vi "Check Expiration.vi"(0 "Vector Charact Result Accessor in":refnum<class "Vector Charact Result Accessor.lvclass">, 11 "error in":errorcluster) -> (4 "Vector Charact Result Accessor out":refnum<class "Vector Charact Result Accessor.lvclass">, 6 "Expired?":bool, 15 "error out":errorcluster)   [LabVIEW 2023, in "RFFixtureCharact.Public.lvlib" / "Vector Charact Result Accessor.lvclass"]
uses:
  Vector Charact Result Accessor.lvclass
  C:/rfcal/AuxTools/STSRFFixtureCharactUtility/Source/Code Modules/Fixture/RMM/Charact Result Accessor/Base/Charact Result Accessor.lvclass
  <vilib>/addons/_RFCalAndCharactDatabase/NI_RFCalAndCharact_Database_API.lvlibp/Characterization/Controls/Type.ctl
  Vector Charact Result Accessor.lvclass/Vector Charact Result Accessor.ctl
  <vilib>/addons/_RFCalAndCharactDatabase/NI_RFCalAndCharact_Database_API.lvlibp/Characterization/Characterization.lvlib
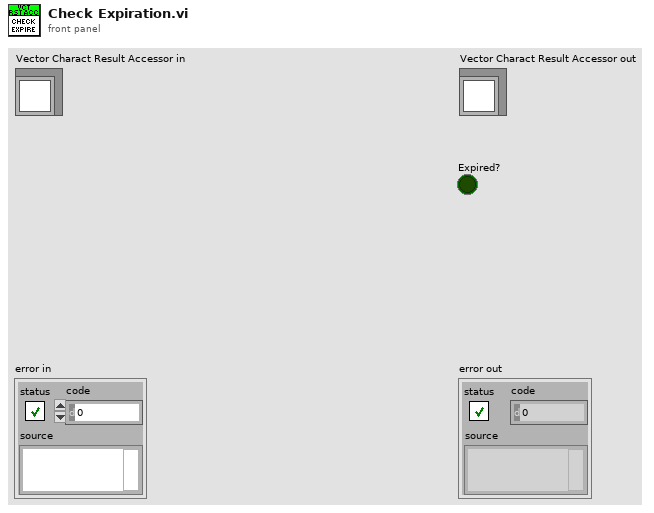
[diagram p1: front panel]
types:
  T1 = typedef "NI_RFCalAndCharact_Database_API.lvlibp/Characterization.lvlib/Type.ctl" = u16
  T2 = typedef "NI_RFCalAndCharact_Database_API.lvlibp/Characterization.lvlib/Path Handle.ctl" = refnum<k24>
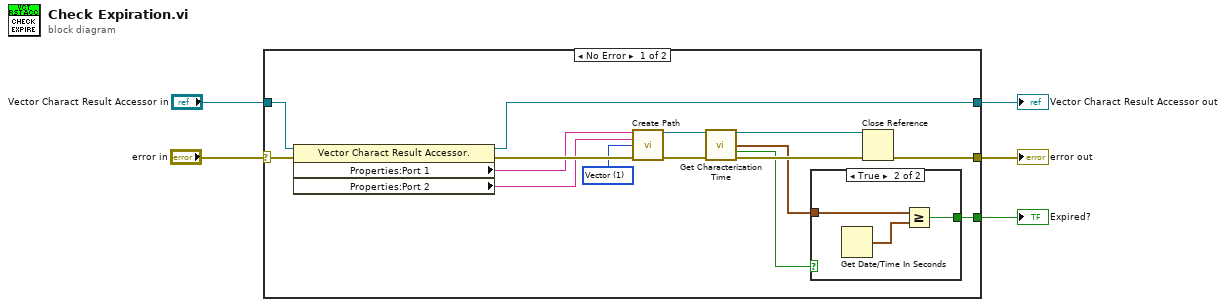
[diagram p0: block diagram]
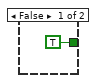
[diagram p2: hidden frame]
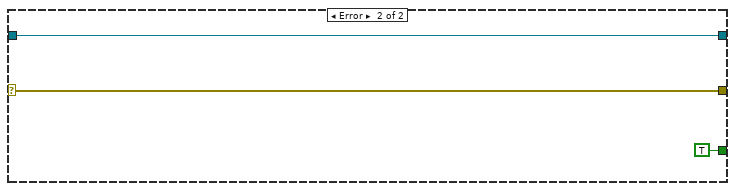
[diagram p3: hidden frame]
diagram:
  n1 = case shown="No Error" "error in" {
    selector: "error in" -> [w15 w26]
    tunnel: "Vector Charact Result Accessor in" -> [w16 w27]
    tunnel: [w10 w27] -> w2
    tunnel: [w9 w26] -> w4
    tunnel: [w6 TRUE] -> w3
    frame No Error {
      w17 = T1 1 items=["Scalar", "Vector"] ("Type")
      n2 = property class="Vector Charact Result Accessor."(reference=w16, error in=w15) -> (reference out=w10:refnum<class "Vector Charact Result Accessor.lvclass">, error out=w20:errorcluster, "Properties:Port 1"=w18:string, "Properties:Port 2"=w19:string)
      n3 = call <vilib>:"Create Path.vi"("Port 1"=w18, "Port 2"=w19, "Type"=w17, "error in"=w20) -> ("Path"=w13:T2, "error out"=w14:errorcluster)  [unwired: 10 in]
      n4 = call <vilib>:"Get Characterization Time.vi"("Path In"=w13, "error in"=w14) -> ("Path Out"=w11:T2, "Characterization Due Time"=w7:timestamp, "Found"=w8:bool, "error out"=w12:errorcluster)  [unwired: 9 in, 1 out]
      n5 = case shown="True" w8 {
        tunnel: w7 -> [_ w24]
        tunnel: [TRUE w22] -> w6
        frame False {
        }
        frame True {
          n6 = Get Date/Time In Seconds() -> (seconds since 1Jan1904=w23:timestamp)
          n7 = Greater Or Equal?(x=w24, y=w23) -> (x >= y?=w22:bool)
        }
      }
      n8 = Close Reference(reference=w11, error in (no error)=w12) -> (error out=w9:errorcluster)
    }
    frame Error {
    }
  }
  "error out" <- w4
  "Vector Charact Result Accessor out" <- w2
  "Expired?" <- w3
